vi "OM3_ShuttleValveControl.vi"() -> ()   [LabVIEW 2015]
uses:
  <vilib>/DAQmx/write.llb/DAQmx Write (Digital Bool 1Line 1Point).vi
  <vilib>/DAQmx/create/channels.llb/DAQmx Create Channel (DO-Digital Output).vi
  <vilib>/DAQmx/miscellaneous.llb/DAQmx Fill In Error Info.vi
panel:
  in  "OM-AE(T)/AM-OE(F)":bool
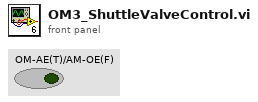
[diagram p1: front panel]
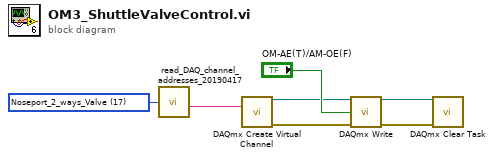
[diagram p0: block diagram]
diagram:
  w1 = u16 17 items=["IR_B_G_LEDs", "L_C_R_Lickometers", "L_R_Lickometers", "[unused]", "R_Water", "L_Water", "Water_Counters", "Analog_Inputs", "Shutter", "Noseport_Hexagonal_Manifold", "Air_Puff", "Lever", "Spouts_Extend", "Spouts_Retract", "Ai_Counter", "Auxiliary_Digital_Inputs", "Sniffing", "Noseport_2_ways_Valve"] ("which channels")
  n1 = call "read_DAQ_channel_addresses_20190417.vi"("which channels"=w1) -> ("myDAQchannels"=w2:string)
  n2 = call-poly <vilib>:"DAQmx Create Virtual Channel.vi"("lines"=w2) -> ("task out"=w3:refnum<k21>, "error out"=w4:errorcluster)  [unwired: 4 in, 9 out]
  n3 = call-poly <vilib>:"DAQmx Write.vi"("task/channels in"=w3, "data"="OM-AE(T)/AM-OE(F)", "error in"=w4) -> ("task out"=w5:refnum<k21>, "error out"=w6:errorcluster)  [unwired: 1 in, 10 out]
  n4 = call <vilib>:"DAQmx Clear Task.vi"("task in"=w5, "error in"=w6) -> ()  [unwired: 14 out]
